vi "niFpgaRegistryGUID.vi"() -> ()   [LabVIEW 2017]
panel:
  in  "CompileWorkerRegistryKey":string="SOFTWARE\\National Instruments\\FPGA CompileWorker\\1.0"
  in  "FarmRegistryKey":string="SOFTWARE\\National Instruments\\NI-Farm\\1.0"
  in  "CloudUrl":string="CompileCloudUrl"
  in  "FarmDll":string="NiFarmClientDll"
  in  "RegistryKey":string="SOFTWARE\\National Instruments\\LabVIEW\\17.0\\AddOns\\FPGA"
  in  "WorkingDirectory":string="WorkingDirectory"
  in  "CompileWorker":string="Path"
  in  "CompileFarm":string="CompileFarmPath"
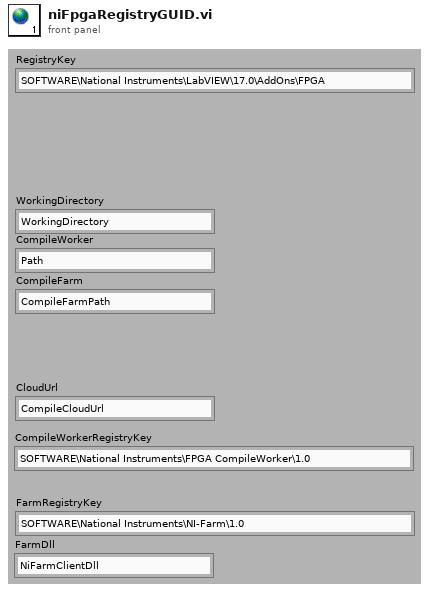
[diagram p1: front panel]
diagram:
